vi "Read Current Ref.vi"(8 "error in (no error)":errorcluster, 11 "Abstract Power Supply in":refnum<class "Abstract Power Supply.lvclass">) -> (0 "error out":errorcluster, 2 "Current Ref":refnum<vi>, 3 "Abstract Power Supply out":refnum<class "Abstract Power Supply.lvclass">)   [LabVIEW 2013, in "Generic Power Supply.lvlib" / "Abstract Power Supply.lvclass"]
uses:
  Abstract Power Supply.lvclass
  Abstract Power Supply.lvclass/Abstract Power Supply.ctl
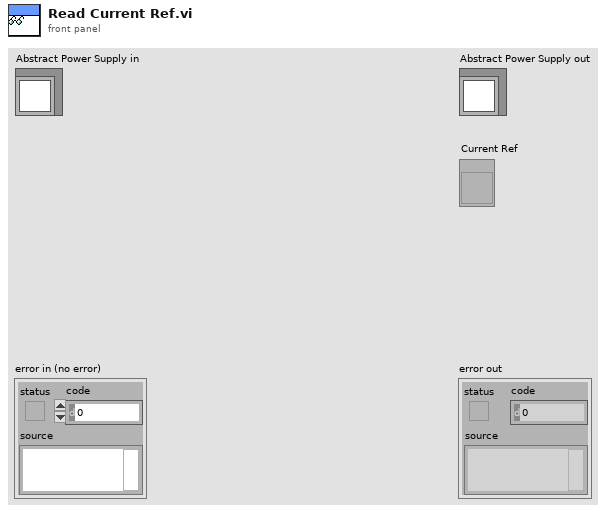
[diagram p1: front panel]
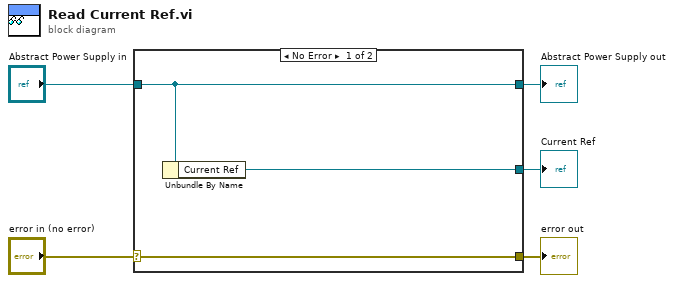
[diagram p0: block diagram]
diagram:
  n1 = case shown="No Error" "error in (no error)" {
    selector: "error in (no error)" -> [w8 w9]
    tunnel: [w8 w9] -> w4
    tunnel: [w7 w10] -> w2
    tunnel: "Abstract Power Supply in" -> [w7 w10]
    tunnel: [w6 _] -> w1
    frame No Error {
      n2 = Unbundle By Name(w7) -> ("Current Ref"=w6:refnum<vi>)
    }
    frame Error {
    }
  }
  "error out" <- w4
  "Abstract Power Supply out" <- w2
  "Current Ref" <- w1
